vi "Climb Immediate.vi"(7 "Description":string, 8 "Command Info In":T2, 10 "Climb States":T1, 11 "Setpoint":dbl) -> (0 "Command Info Out":T2)   [LabVIEW 2023]
doc: "This template is useful for immediate subsystem actions that do not need deadband filtering\n\nBe sure to right-click and select New from Template and save with a new command name."
uses:
  <vilib>/Rock Robotics/WPI/Framework/Command Status Info.ctl
  <vilib>/Rock Robotics/WPI/Framework/Completion Status.ctl
  <vilib>/Rock Robotics/WPI/Framework/Completion Notifier.ctl
  Support Code/Teleop Util/Climb States.ctl
  Implementation/Climb Operations.ctl
  Implementation/Climb Setpoints.ctl
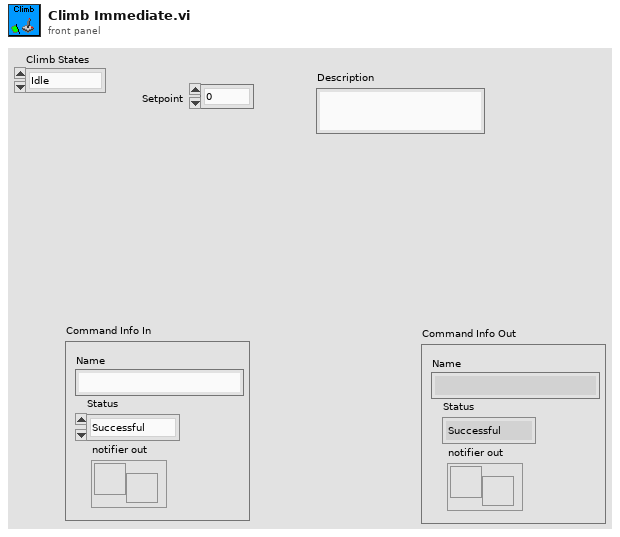
[diagram p1: front panel]
types:
  T1 = typedef "Climb States.ctl" = enum16{"Idle", "Deploy", "Undeploy", "Manual Overrides"}
  T2 = typedef "Command Status Info.ctl" = cluster{"Name":string, "Status":T3, "notifier out":T4}
  T3 = typedef "Completion Status.ctl" = enum16{"Successful", "Aborted", "Incomplete"}
  T4 = typedef "Completion Notifier.ctl" = refnum<notifier>
  T5 = typedef "Climb Operations.ctl" = enum16{"Reserve", "Read Current", "Immediate"}
  T6 = typedef "Climb Setpoints.ctl" = cluster{"Operation":T5, "Setpoint":dbl, "Duration":dbl, "Climb States":T1}
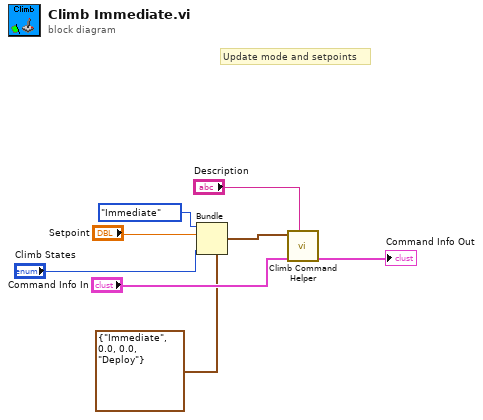
[diagram p0: block diagram]
diagram:
  # "Update mode and setpoints"
  n1 = Bundle(cluster=T6 {"Operation"=enum."Immediate", "Setpoint"=0.0, "Duration"=0.0, "Climb States"=enum."Deploy"} ("SubSystem Data"), "Operation"=Climb_Operations."Immediate", "Setpoint"="Setpoint", "Climb States"="Climb States") -> (w3:T6)  [unwired: 1 in]
  n2 = call "Climb Command Helper.vi"("Description"="Description", "Command Info In"="Command Info In", "SubSystem Data"=w3) -> ("Command Info Out"=→"Command Info Out":T2)  [unwired: 6 in, 2 out]
